vi "dcy05_multimodule.vi"() -> ()   [LabVIEW 2023]
uses:
  parametertype.ctl
  Public/SECoP-action.ctl
  <vilib>/regexp/Match Regular Expression.xnode
  SECoP.lvlib
panel:
  out "error out 2":errorcluster
  out "error out":errorcluster
  out "log":string
  in  "DLL path":path=path "d:/Profile/qfj/Eigene Dateien/LabVIEW-SHALL/64bit"
  in  "stop":bool
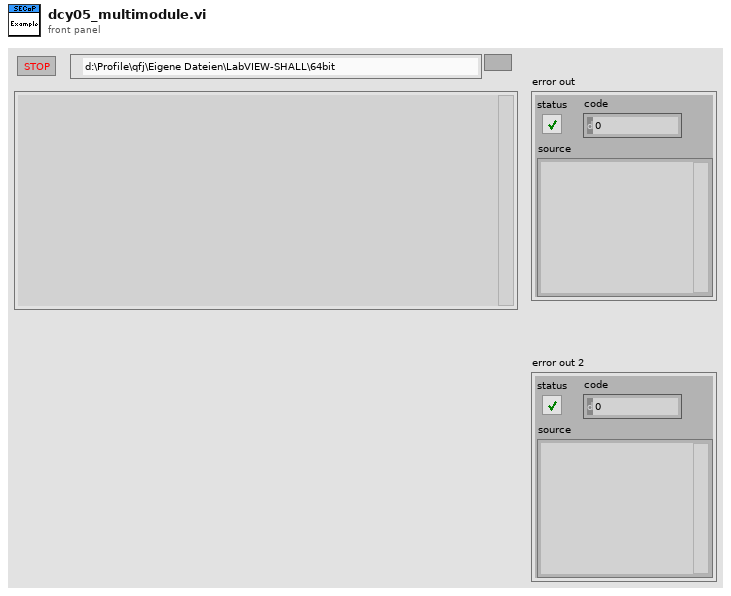
[diagram p1: front panel]
types:
  T1 = typedef "parametertype.ctl" = enum8{"readonly", "readwrite", "command"}
  T2 = cluster{"name":string, "type":T1, "datatype":string, "description":string}[]
  T3 = typedef "SECoP.lvlib/SECoP-libraries.ctl" = cluster{"serverDLL":path, "variantDLL":path, "cleanup_mode":bool}
  T4 = typedef "SECoP.lvlib/SECoP-action.ctl" = enum32{"any action", "read", "change", "do cmd"}
  T5 = cluster{"name":string, "type":T1, "datatype":string, "description":string}
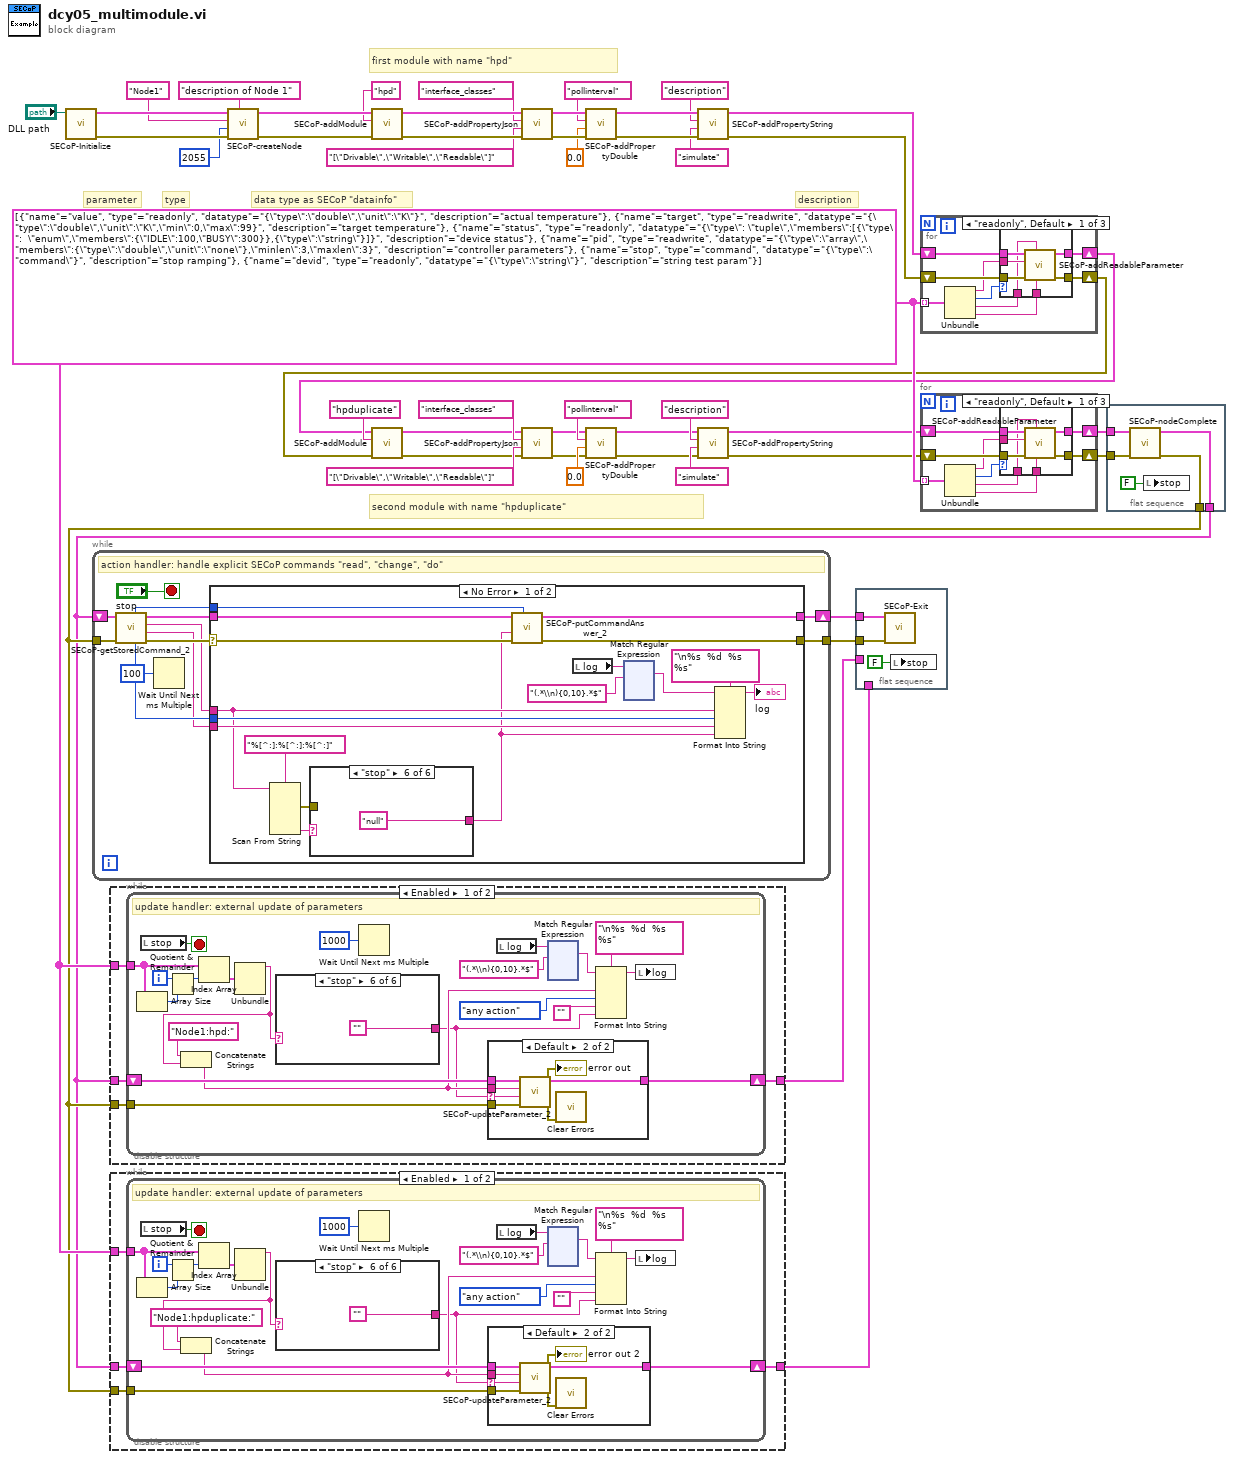
[diagram p0: block diagram]
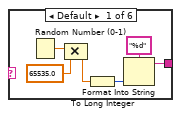
[diagram p3: hidden frame]
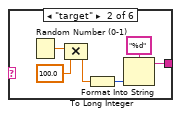
[diagram p4: hidden frame]
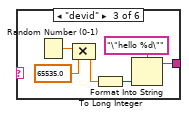
[diagram p5: hidden frame]
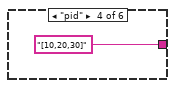
[diagram p6: hidden frame]
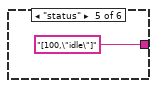
[diagram p7: hidden frame]
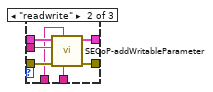
[diagram p9: hidden frame]
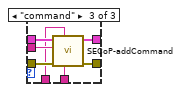
[diagram p10: hidden frame]
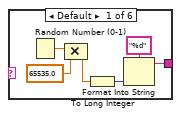
[diagram p12: hidden frame]
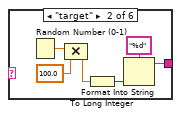
[diagram p13: hidden frame]
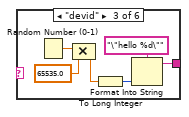
[diagram p14: hidden frame]
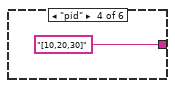
[diagram p15: hidden frame]
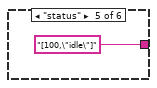
[diagram p16: hidden frame]
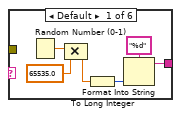
[diagram p18: hidden frame]
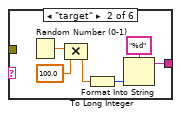
[diagram p19: hidden frame]
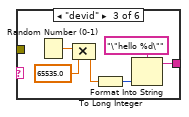
[diagram p20: hidden frame]
diagram:
  w49 = T2 [{"name"="value", "type"=enum."readonly", "datatype"="{\"type\":\"double\",\"unit\":\"K\"}", "description"="actual temperature"}, {"name"="target", "type"=enum."readwrite", "datatype"="{\"type\":\"double\",\"unit\":\"K\",\"min\":0,\"max\":99}", "description"="target temperature"}, {"name"="status", "type"=enum."readonly", "datatype"="{\"type\": \"tuple\",\"members\":[{\"type\":  \"enum\",\"members\":{\"IDLE\":100,\"BUSY\":300}},{\"type\":\"string\"}]}", "description"="device status"}, {"name"="pid", "type"=enum."readwrite", "datatype"="{\"type\":\"array\",\"members\":{\"type\":\"double\",\"unit\":\"none\"},\"minlen\":3,\"maxlen\":3}", "description"="controller parameters"}, {"name"="stop", "type"=enum."command", "datatype"="{\"type\":\"command\"}", "description"="stop ramping"}, {"name"="devid", "type"=enum."readonly", "datatype"="{\"type\":\"string\"}", "description"="string test param"}]
  # "second module with name \"hpduplicate\""
  # "first module with name \"hpd\""
  # "description"
  # "data type as SECoP \"datainfo\""
  # "type"
  # "parameter"
  n1 = call "SECoP-Initialize.vi"("DLL path (in)"="DLL path") -> ("error out"=w44:errorcluster, "DLL path (out)"=w45:T3)  [unwired: 9 in]
  n2 = while {
    shift-right: [w61] -> w33
    shift-left: w2 -> [w59]
    tunnel: w3 -> [w58]
    tunnel: [w51] -> w32
    stop <- "stop" stop-if-true
    # "action handler: handle explicit SECoP commands \"read\", \"change\", \"do\""
    n3 = call "SECoP-getStoredCommand_2.vi"("error in (no error)"=w58, "DLL path (in)"=w59) -> ("error out"=w56:errorcluster, "arguments/setvalue"=w52:string, "command/parameter path"=w53:string, "DLL path (out)"=w57:T3, "action"=w54:T4, "command id"=w55:u64)  [unwired: 4 in]
    n4 = Wait Until Next ms Multiple(millisecond multiple=u32 100) -> ()  [unwired: 1 out]
    n5 = case shown="No Error" w56 {
      selector: w56 -> [w78 w217]
      tunnel: w57 -> [w77 w218]
      tunnel: [w76 w218] -> w61
      tunnel: w55 -> [w75 _]
      tunnel: w53 -> [w66 _]
      tunnel: w52 -> [w72 _]
      tunnel: w54 -> [w73 _]
      tunnel: [w74 w217] -> w51
      frame No Error {
        n6 = Scan From String(format string="%[^:]:%[^:]:%[^:]", input string=w66) -> (error out=w63:errorcluster, output 3=w65:string)  [unwired: 7 in, 2 out]
        n7 = case shown="\"stop\"" w65 {
          tunnel: [w79 w85 w91 "[10,20,30]" "[100,\"idle\"]" "null"] -> w64
          tunnel: w63 -> [_ _ _ _ _ _]
          frame Default {
            n8 = Random Number (0-1)() -> (number: 0 to 1=w81:dbl)
            n9 = Compound Arithmetic op=MULTIPLY(w81, 65535.0 ("value")) -> (w83:dbl)
            n10 = To Long Integer(number=w83) -> (32bit integer=w84:i32)
            n11 = Format Into String(format string="%d", w84) -> (resulting string=w79:string)  [unwired: 2 in, 1 out]
          }
          frame "target" {
            n12 = Random Number (0-1)() -> (number: 0 to 1=w87:dbl)
            n13 = Compound Arithmetic op=MULTIPLY(w87, 100.0 ("value")) -> (w89:dbl)
            n14 = To Long Integer(number=w89) -> (32bit integer=w90:i32)
            n15 = Format Into String(format string="%d", w90) -> (resulting string=w85:string)  [unwired: 2 in, 1 out]
          }
          frame "devid" {
            n16 = Random Number (0-1)() -> (number: 0 to 1=w93:dbl)
            n17 = Compound Arithmetic op=MULTIPLY(w93, 65535.0 ("value")) -> (w95:dbl)
            n18 = To Long Integer(number=w95) -> (32bit integer=w96:i32)
            n19 = Format Into String(format string="\"hello %d\"", w96) -> (resulting string=w91:string)  [unwired: 2 in, 1 out]
          }
          frame "pid" {
          }
          frame "status" {
          }
          frame "stop" {
          }
        }
        n20 = call "SECoP-putCommandAnswer_2.vi"("command id"=w75, "error in (no error)"=w78, "value"=w64, "DLL path (in)"=w77) -> ("error out"=w74:errorcluster, "DLL path (out)"=w76:T3)  [unwired: 6 in]
        n21 = local read "log"() -> (w69:string)
        n22 = xnode "Match Regular Expression"("input string"=w69, "regular expression"="(.*\\n){0,10}.*$") -> ("whole match"=w70:string)  [unwired: 4 in, 4 out]
        n23 = Format Into String(format string="\n%s  %d  %s  %s", initial string=w70, w66, w73, w72, w64) -> (resulting string=→"log":string)  [unwired: 1 in, 1 out]
      }
      frame Error {
      }
    }
  }
  n24 = disable-structure shown="Enabled" {
    disable-tunnel: w3 -> [w222 _]
    disable-tunnel: w49 -> [w221 _]
    disable-tunnel: w2 -> [w220 w389]
    disable-tunnel: [w219 w389] -> w25
    frame Enabled {
      n25 = while {
        tunnel: w222 -> [w224]
        shift-right: [w241] -> w219
        shift-left: w220 -> [w242]
        tunnel: w221 -> [w234]
        i -> [w236]
        stop <- w243 stop-if-true
        # "update handler: external update of parameters"
        n26 = Array Size(array=w234) -> (size(s)=w237:i32)
        n27 = local read "stop"() -> (w243:bool)
        n28 = Quotient & Remainder(x=w236, y=w237) -> (x-y*floor(x/y)=w238:i32)  [unwired: 1 out]
        n29 = Index Array(array=w234, index=w238) -> (element=w235:T5)
        n30 = Unbundle(w235) -> ("name"=w225:string)  [unwired: 3 out]
        n31 = Concatenate Strings("Node1:hpd:" ("string"), w225) -> (w229:string)
        n32 = case shown="\"stop\"" w225 {
          tunnel: [w251 w257 w263 "[10,20,30]" "[100,\"idle\"]" ""] -> w223
          frame Default {
            n33 = Random Number (0-1)() -> (number: 0 to 1=w253:dbl)
            n34 = Compound Arithmetic op=MULTIPLY(w253, 65535.0 ("value")) -> (w255:dbl)
            n35 = To Long Integer(number=w255) -> (32bit integer=w256:i32)
            n36 = Format Into String(format string="%d", w256) -> (resulting string=w251:string)  [unwired: 2 in, 1 out]
          }
          frame "target" {
            n37 = Random Number (0-1)() -> (number: 0 to 1=w259:dbl)
            n38 = Compound Arithmetic op=MULTIPLY(w259, 100.0 ("value")) -> (w261:dbl)
            n39 = To Long Integer(number=w261) -> (32bit integer=w262:i32)
            n40 = Format Into String(format string="%d", w262) -> (resulting string=w257:string)  [unwired: 2 in, 1 out]
          }
          frame "devid" {
            n41 = Random Number (0-1)() -> (number: 0 to 1=w265:dbl)
            n42 = Compound Arithmetic op=MULTIPLY(w265, 65535.0 ("value")) -> (w267:dbl)
            n43 = To Long Integer(number=w267) -> (32bit integer=w268:i32)
            n44 = Format Into String(format string="\"hello %d\"", w268) -> (resulting string=w263:string)  [unwired: 2 in, 1 out]
          }
          frame "pid" {
          }
          frame "status" {
          }
          frame "stop" {
          }
        }
        n45 = Wait Until Next ms Multiple(millisecond multiple=u32 1000) -> ()  [unwired: 1 out]
        n46 = case shown="Default" w223 {
          selector: w223 -> [_ w245]
          tunnel: w242 -> [w244 w250]
          tunnel: [w244 w249] -> w241
          tunnel: w229 -> [_ w248]
          tunnel: w224 -> [_ w247]
          frame "" {
          }
          frame Default {
            n47 = call "SECoP-updateParameter_2.vi"("error in (no error)"=w247, "value"=w245, "parameter name"=w248, "DLL path (in)"=w250) -> ("error out"=w246:errorcluster, "DLL path (out)"=w249:T3)  [unwired: 6 in]
            "error out" <- w246
            n48 = call <vilib>:"Clear Errors.vi"("error in (no error)"=w246) -> ()  [unwired: 5 in, 2 out]
          }
        }
        n49 = local read "log"() -> (w233:string)
        n50 = xnode "Match Regular Expression"("input string"=w233, "regular expression"="(.*\\n){0,10}.*$") -> ("whole match"=w232:string)  [unwired: 4 in, 4 out]
        n51 = Format Into String(format string="\n%s  %d  %s  %s", initial string=w232, w229, SECoP-action."any action" ("input 2"), "", w223) -> (resulting string=w226:string)  [unwired: 1 in, 1 out]
        n52 = local write "log"(w226) -> ()
      }
    }
    frame Disabled {
    }
  }
  n53 = disable-structure shown="Enabled" {
    disable-tunnel: w3 -> [w393 _]
    disable-tunnel: w49 -> [w392 _]
    disable-tunnel: w2 -> [w391 w560]
    disable-tunnel: [w390 w560] -> w1
    frame Enabled {
      n54 = while {
        tunnel: w393 -> [w395]
        shift-right: [w412] -> w390
        shift-left: w391 -> [w413]
        tunnel: w392 -> [w405]
        i -> [w407]
        stop <- w414 stop-if-true
        # "update handler: external update of parameters"
        n55 = Array Size(array=w405) -> (size(s)=w408:i32)
        n56 = local read "stop"() -> (w414:bool)
        n57 = Quotient & Remainder(x=w407, y=w408) -> (x-y*floor(x/y)=w409:i32)  [unwired: 1 out]
        n58 = Index Array(array=w405, index=w409) -> (element=w406:T5)
        n59 = Unbundle(w406) -> ("name"=w396:string)  [unwired: 3 out]
        n60 = Concatenate Strings("Node1:hpduplicate:" ("string"), w396) -> (w400:string)
        n61 = case shown="\"stop\"" w396 {
          tunnel: [w422 w428 w434 "[10,20,30]" "[100,\"idle\"]" ""] -> w394
          frame Default {
            n62 = Random Number (0-1)() -> (number: 0 to 1=w424:dbl)
            n63 = Compound Arithmetic op=MULTIPLY(w424, 65535.0 ("value")) -> (w426:dbl)
            n64 = To Long Integer(number=w426) -> (32bit integer=w427:i32)
            n65 = Format Into String(format string="%d", w427) -> (resulting string=w422:string)  [unwired: 2 in, 1 out]
          }
          frame "target" {
            n66 = Random Number (0-1)() -> (number: 0 to 1=w430:dbl)
            n67 = Compound Arithmetic op=MULTIPLY(w430, 100.0 ("value")) -> (w432:dbl)
            n68 = To Long Integer(number=w432) -> (32bit integer=w433:i32)
            n69 = Format Into String(format string="%d", w433) -> (resulting string=w428:string)  [unwired: 2 in, 1 out]
          }
          frame "devid" {
            n70 = Random Number (0-1)() -> (number: 0 to 1=w436:dbl)
            n71 = Compound Arithmetic op=MULTIPLY(w436, 65535.0 ("value")) -> (w438:dbl)
            n72 = To Long Integer(number=w438) -> (32bit integer=w439:i32)
            n73 = Format Into String(format string="\"hello %d\"", w439) -> (resulting string=w434:string)  [unwired: 2 in, 1 out]
          }
          frame "pid" {
          }
          frame "status" {
          }
          frame "stop" {
          }
        }
        n74 = Wait Until Next ms Multiple(millisecond multiple=u32 1000) -> ()  [unwired: 1 out]
        n75 = case shown="Default" w394 {
          selector: w394 -> [_ w416]
          tunnel: w413 -> [w415 w421]
          tunnel: [w415 w420] -> w412
          tunnel: w400 -> [_ w419]
          tunnel: w395 -> [_ w418]
          frame "" {
          }
          frame Default {
            n76 = call "SECoP-updateParameter_2.vi"("error in (no error)"=w418, "value"=w416, "parameter name"=w419, "DLL path (in)"=w421) -> ("error out"=w417:errorcluster, "DLL path (out)"=w420:T3)  [unwired: 6 in]
            "error out 2" <- w417
            n77 = call <vilib>:"Clear Errors.vi"("error in (no error)"=w417) -> ()  [unwired: 5 in, 2 out]
          }
        }
        n78 = local read "log"() -> (w404:string)
        n79 = xnode "Match Regular Expression"("input string"=w404, "regular expression"="(.*\\n){0,10}.*$") -> ("whole match"=w403:string)  [unwired: 4 in, 4 out]
        n80 = Format Into String(format string="\n%s  %d  %s  %s", initial string=w403, w400, SECoP-action."any action" ("input 2"), "", w394) -> (resulting string=w397:string)  [unwired: 1 in, 1 out]
        n81 = local write "log"(w397) -> ()
      }
    }
    frame Disabled {
    }
  }
  n82 = call "SECoP-createNode.vi"("description"="description of Node 1", "error in (no error)"=w44, "TCP port"=u16 2055, "node id"="Node1" ("id"), "DLL path (in)"=w45) -> ("error out"=w39:errorcluster, "DLL path (out)"=w43:T3)  [unwired: 5 in]
  n83 = call "SECoP-addModule.vi"("error in (no error)"=w39, "module name"="hpd" ("name"), "DLL path (in)"=w43) -> ("error out"=w36:errorcluster, "DLL path (out)"=w37:T3)  [unwired: 7 in]
  n84 = call "SECoP-addPropertyJson.vi"("error in (no error)"=w36, "property value"="[\"Drivable\",\"Writable\",\"Readable\"]" ("name"), "property name"="interface_classes" ("name"), "DLL path (in)"=w37) -> ("error out"=w28:errorcluster, "DLL path (out)"=w29:T3)  [unwired: 6 in]
  n85 = call "SECoP-addPropertyDouble.vi"("error in (no error)"=w28, "property value"=0.0, "property name"="pollinterval", "DLL path (in)"=w29) -> ("error out"=w48:errorcluster, "DLL path (out)"=w47:T3)  [unwired: 6 in]
  n86 = call "SECoP-addPropertyString.vi"("error in (no error)"=w48, "property value"="simulate" ("name"), "property name"="description" ("name"), "DLL path (in)"=w47) -> ("error out"=w23:errorcluster, "DLL path (out)"=w24:T3)  [unwired: 6 in]
  n87 = flat-sequence {
    tunnel: w33 -> [w562]
    tunnel: w32 -> [w561]
    tunnel: w25 -> [_]
    tunnel: w1 -> [_]
    frame #0 {
      n88 = call "SECoP-Exit.vi"("error in (no error)"=w561, "DLL path (in)"=w562) -> ()  [unwired: 9 in, 1 out]
      n89 = local write "stop"(FALSE) -> ()
    }
  }
  n90 = for {
    tunnel: w49 -> [w568] mode=indexing
    shift-right: [w565] -> w6
    shift-left: w24 -> [w571]
    shift-right: [w564] -> w5
    shift-left: w23 -> [w570]
    n91 = Unbundle(w568) -> ("name"=w569:string, "type"=w572:T1, "datatype"=w567:string, "description"=w566:string)
    n92 = case shown="\"readonly\", Default" w572 {
      tunnel: w569 -> [w577 w586 w593]
      tunnel: w571 -> [w579 w585 w592]
      tunnel: [w578 w584 w591] -> w565
      tunnel: [w575 w582 w589] -> w564
      tunnel: w570 -> [w576 w583 w590]
      tunnel: w567 -> [w574 w580 w588]
      tunnel: w566 -> [w573 w581 w587]
      frame "readonly", Default {
        n93 = call "SECoP-addReadableParameter.vi"("description"=w573, "datainfo"=w574, "error in (no error)"=w576, "parameter name"=w577, "DLL path (in)"=w579) -> ("error out"=w575:errorcluster, "DLL path (out)"=w578:T3)  [unwired: 5 in]
      }
      frame "readwrite" {
        n94 = call "SECoP-addWritableParameter.vi"("description"=w581, "datainfo"=w580, "error in (no error)"=w583, "parameter name"=w586, "DLL path (in)"=w585) -> ("error out"=w582:errorcluster, "DLL path (out)"=w584:T3)  [unwired: 5 in]
      }
      frame "command" {
        n95 = call "SECoP-addCommand.vi"("description"=w587, "datainfo"=w588, "error in (no error)"=w590, "command name"=w593, "DLL path (in)"=w592) -> ("error out"=w589:errorcluster, "DLL path (out)"=w591:T3)  [unwired: 5 in]
      }
    }
  }
  n96 = call "SECoP-addModule.vi"("error in (no error)"=w5, "module name"="hpduplicate" ("name"), "DLL path (in)"=w6) -> ("error out"=w14:errorcluster, "DLL path (out)"=w13:T3)  [unwired: 7 in]
  n97 = call "SECoP-addPropertyJson.vi"("error in (no error)"=w14, "property value"="[\"Drivable\",\"Writable\",\"Readable\"]" ("name"), "property name"="interface_classes" ("name"), "DLL path (in)"=w13) -> ("error out"=w20:errorcluster, "DLL path (out)"=w19:T3)  [unwired: 6 in]
  n98 = call "SECoP-addPropertyDouble.vi"("error in (no error)"=w20, "property value"=0.0, "property name"="pollinterval", "DLL path (in)"=w19) -> ("error out"=w10:errorcluster, "DLL path (out)"=w11:T3)  [unwired: 6 in]
  n99 = call "SECoP-addPropertyString.vi"("error in (no error)"=w10, "property value"="simulate" ("name"), "property name"="description" ("name"), "DLL path (in)"=w11) -> ("error out"=w7:errorcluster, "DLL path (out)"=w8:T3)  [unwired: 6 in]
  n100 = for {
    tunnel: w49 -> [w598] mode=indexing
    shift-right: [w595] -> w9
    shift-left: w8 -> [w601]
    shift-right: [w594] -> w4
    shift-left: w7 -> [w600]
    n101 = Unbundle(w598) -> ("name"=w599:string, "type"=w602:T1, "datatype"=w597:string, "description"=w596:string)
    n102 = case shown="\"readonly\", Default" w602 {
      tunnel: w599 -> [w607 w616 w623]
      tunnel: w601 -> [w609 w615 w622]
      tunnel: [w608 w614 w621] -> w595
      tunnel: [w605 w612 w619] -> w594
      tunnel: w600 -> [w606 w613 w620]
      tunnel: w597 -> [w604 w610 w618]
      tunnel: w596 -> [w603 w611 w617]
      frame "readonly", Default {
        n103 = call "SECoP-addReadableParameter.vi"("description"=w603, "datainfo"=w604, "error in (no error)"=w606, "parameter name"=w607, "DLL path (in)"=w609) -> ("error out"=w605:errorcluster, "DLL path (out)"=w608:T3)  [unwired: 5 in]
      }
      frame "readwrite" {
        n104 = call "SECoP-addWritableParameter.vi"("description"=w611, "datainfo"=w610, "error in (no error)"=w613, "parameter name"=w616, "DLL path (in)"=w615) -> ("error out"=w612:errorcluster, "DLL path (out)"=w614:T3)  [unwired: 5 in]
      }
      frame "command" {
        n105 = call "SECoP-addCommand.vi"("description"=w617, "datainfo"=w618, "error in (no error)"=w620, "command name"=w623, "DLL path (in)"=w622) -> ("error out"=w619:errorcluster, "DLL path (out)"=w621:T3)  [unwired: 5 in]
      }
    }
  }
  n106 = flat-sequence {
    tunnel: w9 -> [w627]
    tunnel: w4 -> [w626]
    tunnel: [w624] -> w2
    tunnel: [w625] -> w3
    frame #0 {
      n107 = call "SECoP-nodeComplete.vi"("error in (no error)"=w626, "DLL path (in)"=w627) -> ("error out"=w625:errorcluster, "DLL path (out)"=w624:T3)  [unwired: 8 in]
      n108 = local write "stop"(FALSE) -> ()
    }
  }
